vi "Monitor (Sub vi).vi"(0 "VISA Refnum in":refnum<visa-resource-name>, 1 "Range":T2(ring), 2 "Response":enum16{"FAST", "STD", "SLOW"}(ring), 3 "Auto Zero Pos":enum16{"0", "5", "10", "50", "100"}(ring), 4 "Integrator Output\n Range":T1(ring), 5 "error in (no error)":errorcluster, 6 "Auto Zero":enum16{"AUTO", "MANUAL", "HOLD"}(ring), 7 "Signal Filter":enum16{"Time Acc", "CR", "Digital"}(ring), 8 "Polarity":enum16{"Plus", "Minus"}(ring), 9 "Program File No.":u32 max=9 step=1, 10 "Sampling Time (ms)":u32=250, 11 "Wavelength (nm)":u32=190 min=190 max=600 step=1) -> (14 "VISA Refnum out":refnum<visa-resource-name>, 15 "Absorbance (ABU)":dbl, 16 "Waveform Chart":ext(graph), 17 "String out":string, 19 "error out":errorcluster)   [LabVIEW 2020, in "Jasco UV.lvlib"]
uses:
  Jasco UV.lvlib
  Action-Status/Operations.ctl
  Data/Read Controls.ctl
  e6f6fdae-fb0d-46c7-9a14-e00745f985dd.vi
  5cc56714-22f3-4ff6-886f-b8f8bffa08ae.vi
  720c64e1-63cb-4cbf-bff6-f2c58a61a871.vi
  1fe2776a-1b09-4367-999f-5bdc5cb06da5.vi
  cf873e07-79d1-4aff-953a-e1dc5794681d.vi
  7b48cdc8-4b13-4ea8-a860-c4d74ff25f47.vi
  374b93a3-ebf8-4097-ae14-143701f66a32.vi
  672fa7bb-6108-42d6-9f17-8afbc275381c.vi
  8b855db6-c1f8-49de-b381-13d5f98214f5.vi
  <userlib>/_OpenG.lib/string/string.llb/Trim Whitespace (String)__ogtk.vi
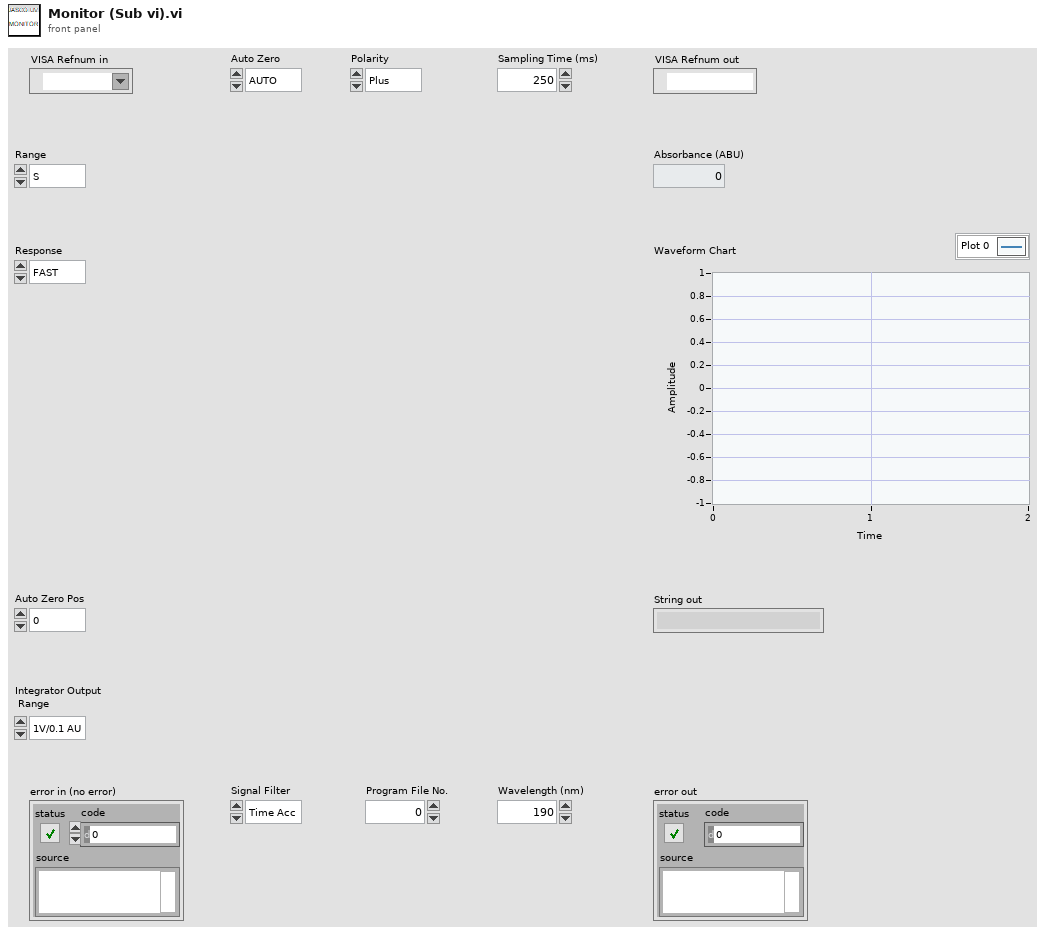
[diagram p1: front panel]
types:
  T1 = enum16{"1V/0.1 AU", "1V/1.0 AU", "1V/2.0 AU", "1V/3.0 AU"}
  T2 = enum16{"S", "2.56", "1.28", "0.64", "0.32", "0.16", "0.08", "0.04", "0.02", "0.01", "0.005", "0.0025", "0.00125", "0.0005"}
  T3 = typedef "Jasco UV.lvlib/Read Controls.ctl" = string
  T4 = typedef "Jasco UV.lvlib/Operations.ctl" = string
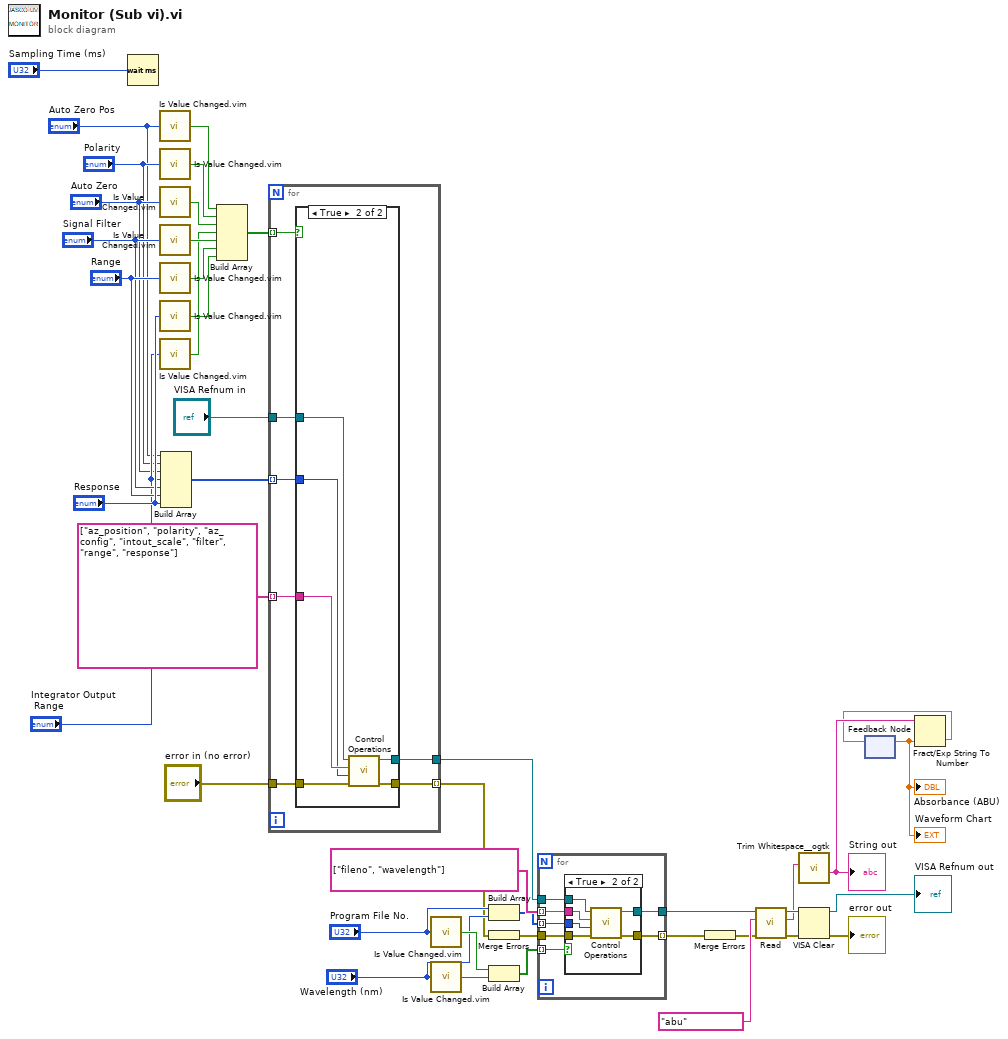
[diagram p0: block diagram]
diagram:
  n1 = Wait (ms)(milliseconds to wait="Sampling Time (ms)") -> ()  [unwired: 1 out]
  n2 = call "Is Value Changed.vim"("value"="Auto Zero Pos") -> ("changed or first call?"=w22:bool)
  n3 = call "Is Value Changed.vim"("value"="Polarity") -> ("changed or first call?"=w23:bool)
  n4 = call "Is Value Changed.vim"("value"="Auto Zero") -> ("changed or first call?"=w24:bool)
  n5 = call "Is Value Changed.vim"("value"="Signal Filter") -> ("changed or first call?"=w26:bool)
  n6 = call "Is Value Changed.vim"("value"="Range") -> ("changed or first call?"=w27:bool)
  n7 = call "Is Value Changed.vim"("value"="Response") -> ("changed or first call?"=w28:bool)
  n8 = call "Is Value Changed.vim"("value"="Integrator Output\n Range") -> ("changed or first call?"=w25:bool)
  n9 = Build Array("Auto Zero Pos", "Polarity", "Auto Zero", "Integrator Output\n Range", "Signal Filter", "Range", "Response") -> (w14:u16[])
  n10 = Build Array(w22, w23, w24, w25, w26, w27, w28) -> (w29:bool[])
  n11 = for {
    tunnel: "VISA Refnum in" -> [w49]
    tunnel: w14 -> [w44] mode=indexing
    tunnel: T4[] ["az_position", "polarity", "az_config", "intout_scale", "filter", "range", "response"] -> [w48] mode=indexing
    tunnel: "error in (no error)" -> [w47]
    tunnel: [w46] -> w7
    tunnel: [w45] -> w4 mode=indexing
    tunnel: w29 -> [w43] mode=indexing
    n12 = case shown="True" w43 {
      tunnel: w49 -> [w50 w57]
      tunnel: w48 -> [_ w56]
      tunnel: w44 -> [_ w55]
      tunnel: w47 -> [w51 w54]
      tunnel: [w50 w53] -> w46
      tunnel: [w51 w52] -> w45
      frame False {
      }
      frame True {
        n13 = call "Control Operations.vi"("error in (no error)"=w54, "Value"=w55, "Command"=w56, "VISA resource name"=w57) -> ("error out"=w52:errorcluster, "VISA resource name out"=w53:refnum<visa-resource-name>)  [unwired: 6 in]
      }
    }
  }
  n14 = call "Is Value Changed.vim"("value"="Program File No.") -> ("changed or first call?"=w33:bool)
  n15 = call "Is Value Changed.vim"("value"="Wavelength (nm)") -> ("changed or first call?"=w32:bool)
  n16 = Build Array("Program File No.", "Wavelength (nm)") -> (w5:u32[])
  n17 = Merge Errors(w4) -> (w8:errorcluster)
  n18 = Build Array(w33, w32) -> (w34:bool[])
  n19 = for {
    tunnel: w7 -> [w64]
    tunnel: w5 -> [w58] mode=indexing
    tunnel: T4[] ["fileno", "wavelength"] -> [w63] mode=indexing
    tunnel: w8 -> [w62]
    tunnel: [w61] -> w10
    tunnel: [w60] -> w9 mode=indexing
    tunnel: w34 -> [w59] mode=indexing
    n20 = case shown="True" w59 {
      tunnel: w64 -> [w65 w72]
      tunnel: w63 -> [_ w71]
      tunnel: w58 -> [_ w70]
      tunnel: w62 -> [w66 w69]
      tunnel: [w65 w68] -> w61
      tunnel: [w66 w67] -> w60
      frame False {
      }
      frame True {
        n21 = call "Control Operations.vi"("error in (no error)"=w69, "Value"=w70, "Command"=w71, "VISA resource name"=w72) -> ("error out"=w67:errorcluster, "VISA resource name out"=w68:refnum<visa-resource-name>)  [unwired: 6 in]
      }
    }
  }
  n22 = Merge Errors(w9) -> (w11:errorcluster)
  n23 = call "Read.vi"("error in (no error)"=w11, "Command"=T3 "abu", "VISA resource name"=w10) -> ("error out"=w41:errorcluster, "read buffer"=w37:string, "VISA resource name out"=w39:refnum<visa-resource-name>)  [unwired: 6 in]
  n24 = call-poly <userlib>:"Trim Whitespace__ogtk.vi"("String in"=w37) -> ("String out"=w38:string)  [unwired: 6 in]
  "String out" <- w38
  n25 = VISA Clear(VISA resource name=w39, error in (no error)=w41) -> (VISA resource name out=→"VISA Refnum out":refnum<visa-resource-name>, error out=→"error out":errorcluster)
  n26 = feedback #1() -> (w36:ext)  [unwired: 1 in]
  "Absorbance (ABU)" <- w36
  "Waveform Chart" <- w36
  n27 = Fract/Exp String To Number(string=w38, default (0 dbl)=w36) -> (number=w35:ext)  [unwired: 2 in, 1 out]
  n28 = feedback-in #1(w35) -> ()
